vi "ROI entry-ROI fitting dialogue.vi"(11 "Frame size":cluster{"Old":T1, "New":T1} {"Old" items=["100X100"=100, "128X128"=128, "200X200"=200, "256X256"=256, "512X512"=512, "1024x1024"=1024, "2048x2048"=2048]; "New" items=["100X100"=100, "128X128"=128, "200X200"=200, "256X256"=256, "512X512"=512, "1024x1024"=1024, "2048x2048"=2048]}) -> (3 "Cancelled (Left button pressed)":bool)   [LabVIEW 2013]
uses:
  Typedefs/Frame Size.ctl
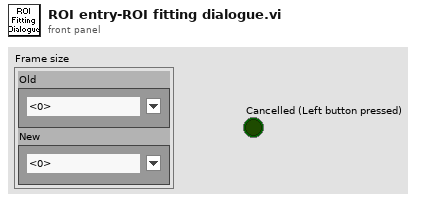
[diagram p1: front panel]
types:
  T1 = typedef "Frame Size.ctl" = u16
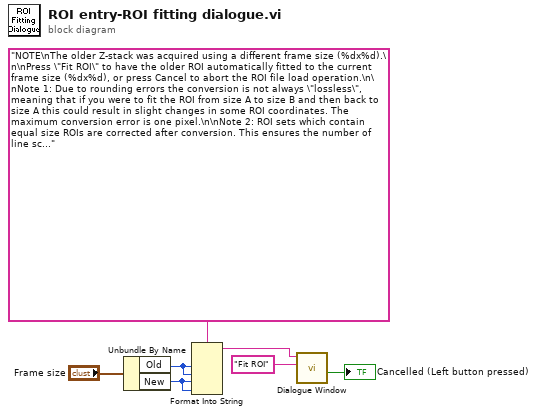
[diagram p0: block diagram]
diagram:
  n1 = Unbundle By Name("Frame size") -> ("Old"=w3:T1, "New"=w2:T1)
  n2 = Format Into String(format string="NOTE\nThe older Z-stack was acquired using a different frame size (%dx%d).\n\nPress \"Fit ROI\" to have the older ROI automatically fitted to the current frame size (%dx%d), or press Cancel to abort the ROI file load operation.\n\nNote 1: Due to rounding errors the conversion is not always \"lossless\", meaning that if you were to fit the ROI from size A to size B and then back to size A this could result in slight changes in some ROI coordinates. The maximum conversion error is one pixel.\n\nNote 2: ROI sets which contain equal size ROIs are corrected after conversion. This ensures the number of line scans each ROI consists of after conversion, is still equal with that of all other ROIs which had equal number of line scans in the original ROI set.\n" ("Message string"), w3, w3, w2, w2) -> (resulting string=w1:string)  [unwired: 2 in, 1 out]
  n3 = call "Dialogue Window.vi"("Caption-Right button (OK)"="Fit ROI", "Message string"=w1) -> ("Cancelled (Left button pressed)"=→"Cancelled (Left button pressed)":bool)  [unwired: 7 in, 2 out]
